vi "Execute Msg Or Recurse.vi"(7 "Actor in":refnum<class "Actor.lvclass">, 10 "Msg":refnum<class "Msg.lvclass">) -> (0 "Error out":errorcluster, 2 "Msg Output":refnum<class "Msg Output.lvclass">, 5 "Actor out":refnum<class "Actor.lvclass">)   [LabVIEW 2025, in "jettl.lvlib"]
uses:
  jettl.lvlib
  Msg/Msg.lvclass
  Actor/Actor.lvclass
  Msg Output/Msg Output.lvclass
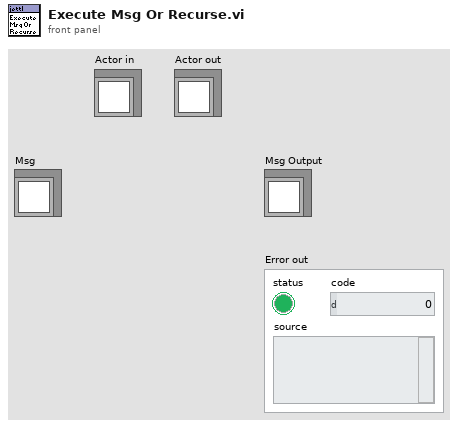
[diagram p1: front panel]
types:
  T1 = typedef "jettl.lvlib/Msg Set.ctl" = set{refnum<class "Msg.lvclass">}
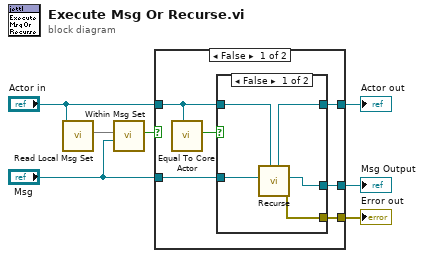
[diagram p0: block diagram]
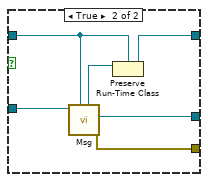
[diagram p3: hidden frame]
diagram:
  n1 = call-dynamic "Read Local Msg Set.vi"("Actor in"="Actor in") -> ("Local Msg Set"=w4:T1)  [unwired: 10 in]
  n2 = call "Within Msg Set.vi"("Msg"="Msg", "Msg Set"=w4) -> ("Within Msg Set"=w7:bool)  [unwired: 9 in]
  n3 = case shown="False" w7 {
    tunnel: "Actor in" -> [w9 w23]
    tunnel: [w11 w22] -> w2
    tunnel: "Msg" -> [w13 w25]
    tunnel: [w12 w21] -> w5
    tunnel: [w10 w20] -> w1
    frame False {
      n4 = call "Equal To Core Actor.vi"("Actor"=w9) -> ("Core Actor"=w8:bool)  [unwired: 10 in]
      n5 = case shown="False" w8 {
        tunnel: w13 -> [w16 _]
        tunnel: [w15 _] -> w12
        tunnel: w9 -> [w18 w19]
        tunnel: [w17 w19] -> w11
        tunnel: [w14 _] -> w10
        frame False {
          n6 = call "Recurse.vi"("Actor in"=w18, "Msg"=w16) -> ("Error out"=w15:errorcluster, "Msg Output"=w14:refnum<class "Msg Output.lvclass">, "Actor out"=w17:refnum<class "Actor.lvclass">)  [unwired: 7 in]
        }
        frame True {
          # "This is the core, do nothing."
        }
      }
    }
    frame True {
      n7 = call-dynamic "Msg.vi"("Actor in"=w23, "Msg in"=w25) -> ("Error out"=w21:errorcluster, "Msg Output"=w20:refnum<class "Msg Output.lvclass">, "Actor out"=w24:refnum<class "Actor.lvclass">)  [unwired: 7 in]
      n8 = Preserve Run-Time Class(object in=w24, 2:w23) -> (object out=w22:refnum<class "Actor.lvclass">)  [unwired: 1 in, 1 out]
    }
  }
  "Error out" <- w5
  "Actor out" <- w2
  "Msg Output" <- w1
